vi "Get DLL Version.vi"(8 "error in (no error)":errorcluster, 11 "USBTransferNfoPtr":u32) -> (0 "error out":errorcluster, 2 "function return":string, 3 "USBTransferNfoPtr out":u32)   [LabVIEW 2017, in "ZBOX_IS.lvlib"]
doc: "char *GetDLLVersion(unsigned long *USBTransferNfoPtr);"
uses:
  ZBOX_IS.lvlib
  PicometerCtrl.dll
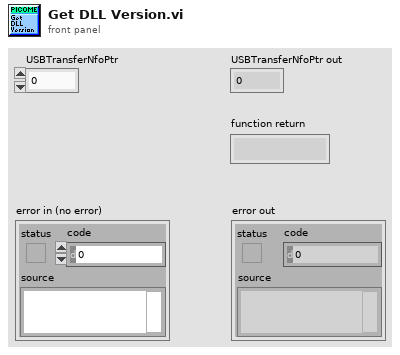
[diagram p1: front panel]
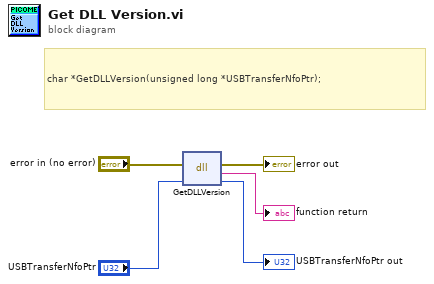
[diagram p0: block diagram]
diagram:
  # "char *GetDLLVersion(unsigned long *USBTransferNfoPtr);"
  n1 = dll-call lib="C:/Users/Marek/Desktop/Quadra Software Package v1.1/LabView/Zbox_is/Public/Configure/Low Level/__DLL_functions/PicometerCtrl.dll" fn="GetDLLVersion"(error in="error in (no error)", "USBTransferNfoPtr"="USBTransferNfoPtr") -> (error out=→"error out":errorcluster, "return type"=→"function return":string, "USBTransferNfoPtr"=→"USBTransferNfoPtr out":u32)  [unwired: 2 in, 1 out]
